vi "heartbeatWrite.vi"() -> ()   [LabVIEW 2018, in "MotorControllerClass.lvclass"]
uses:
  BMS/MotorControllerClass.lvclass
panel:
  out "MotorController Class out":refnum<class "MotorControllerClass.lvclass">
  out "interface object out":refnum<k20>
  in  "interface object in":refnum<k20>
  out "error out":errorcluster
  in  "error in (no error)":errorcluster
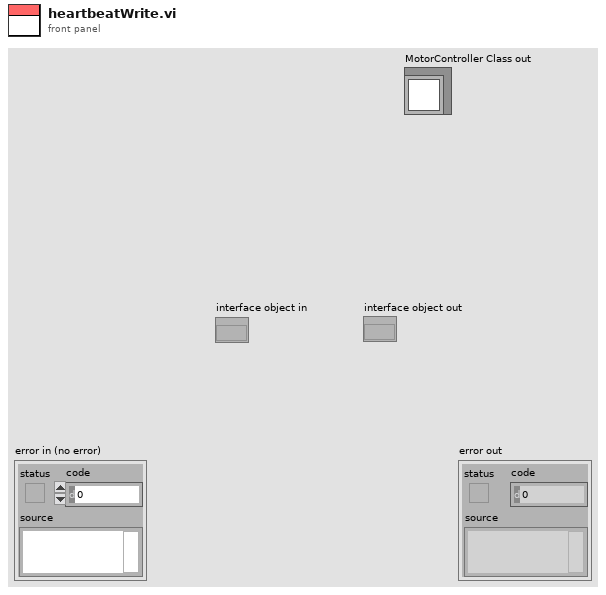
[diagram p1: front panel]
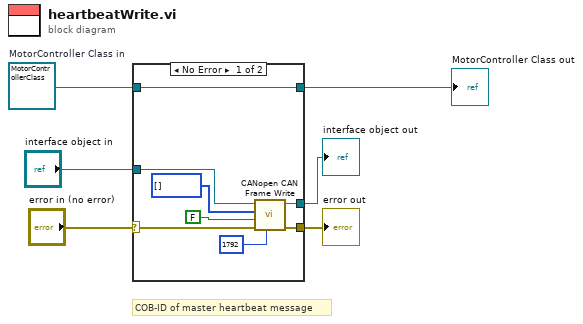
[diagram p0: block diagram]
diagram:
  w2 = refnum<class "MotorControllerClass.lvclass"> refnum  # MotorController Class in
  # "COB-ID of master heartbeat message"
  n1 = case shown="No Error" "error in (no error)" {
    selector: "error in (no error)" -> [w11 w17]
    tunnel: [w9 w17] -> w5
    tunnel: [w14 w16] -> w1
    tunnel: w2 -> [w14 w16]
    tunnel: "interface object in" -> [w13 w15]
    tunnel: [w7 w15] -> w3
    frame No Error {
      n2 = call <vilib>:"CANopen CAN Frame Write.vi"("COB-ID (0)"=u32 1792, "error in (no error)"=w11, "RTR? (F)"=FALSE, "CAN message data"=u8[] [], "interface object  in"=w13) -> ("error out"=w9:errorcluster, "interface object out"=w7:refnum<k20>)  [unwired: 5 in]
    }
    frame Error {
    }
  }
  "error out" <- w5
  "interface object out" <- w3
  "MotorController Class out" <- w1
